vi "Parse Value.vi"(0 "JSON String":string, 5 "Index In":i32, 11 "error in (no error)":errorcluster) -> (4 "Variant out":variant, 6 "Index Out":i32, 15 "error out":errorcluster)   [LabVIEW 2017, in "Variant JSON API.lvlib"]
uses:
  Variant JSON API.lvlib
  Errors.ctl
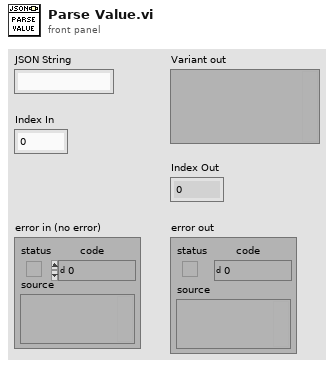
[diagram p1: front panel]
types:
  T1 = typedef "Variant JSON API.lvlib/Errors.ctl" = enum16{"No key", "Key path type", "Array OOB", "Type Mismatch", "Invalid Token", "Invalid Value"}
  T2 = typedef "Variant JSON API.lvlib/Token Type.ctl" = enum16{"NONE", "CURLY_OPEN", "CURLY_CLOSE", "SQUARED_OPEN", "SQUARED_CLOSE", "COLON", "COMMA", "STRING", "NUMBER", "TRUE", "FALSE", "NULL"}
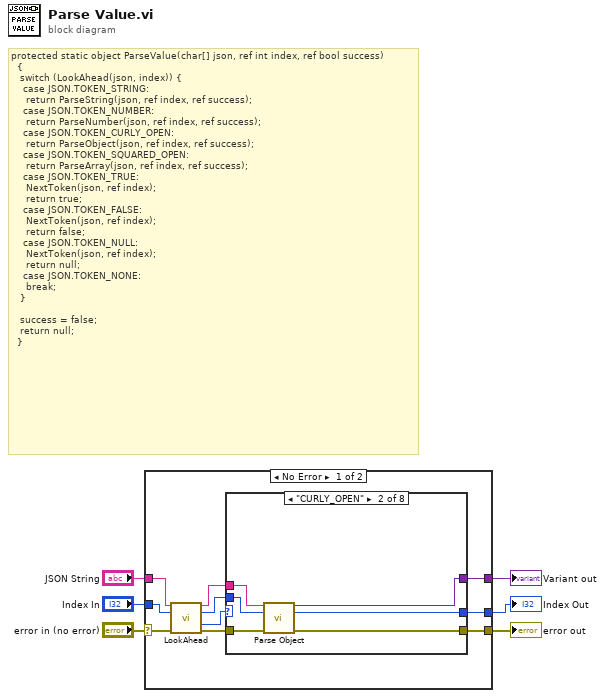
[diagram p0: block diagram]
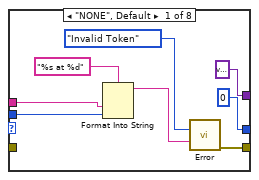
[diagram p2: hidden frame]
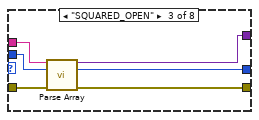
[diagram p3: hidden frame]
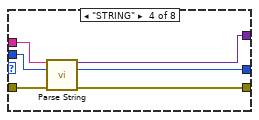
[diagram p4: hidden frame]
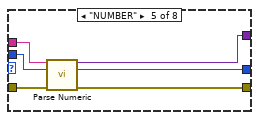
[diagram p5: hidden frame]
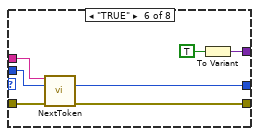
[diagram p6: hidden frame]
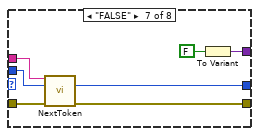
[diagram p7: hidden frame]
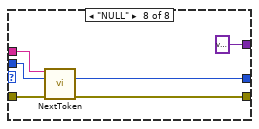
[diagram p8: hidden frame]
diagram:
  # "protected static object ParseValue(char[] json, ref int index, ref bool success)\n\t\t{\n\t\t\tswitch (LookAhead(json, index)) {\n\t\t\t\tcase JSON.TOKEN_STRING:\n\t\t\t\t\treturn ParseString(json, ref index, ref success);\n\t\t\t\tcase JSON.TOKEN_NUMBER:\n\t\t\t\t\treturn ParseNumber(json, ref index, ref success);\n\t\t\t\tcase JSON.TOKEN_CURLY_OPEN:\n\t\t\t\t\treturn ParseObject(json, ref index, ref success);\n\t\t\t\tcase JSON.TOKEN_SQUARED_OPEN:\n\t\t\t\t\treturn ParseArray(json, ref index, ref success);\n\t\t\t\tcase JSON.TOKEN_TRUE:\n\t\t\t\t\tNextToken(json, ref index);\n\t\t\t\t\treturn true;\n\t\t\t\tcase JSON.TOKEN_FALSE:\n\t\t\t\t\tNextToken(json, ref index);\n\t\t\t\t\treturn false;\n\t\t\t\tcase JSON.TOKEN_NULL:\n\t\t\t\t\tNextToken(json, ref index);\n\t\t\t\t\treturn null;\n\t\t\t\tcase JSON.TOKEN_NONE:\n\t\t\t\t\tbreak;\n\t\t\t}\n\n\t\t\tsuccess = false;\n\t\t\treturn null;\n\t\t}"
  n1 = case shown="No Error" "error in (no error)" {
    selector: "error in (no error)" -> [w16 w69]
    tunnel: [w14 w69] -> w5
    tunnel: "JSON String" -> [w10 _]
    tunnel: "Index In" -> [w9 _]
    tunnel: [w8 _] -> w1
    tunnel: [w7 _] -> w2
    frame No Error {
      n2 = call "LookAhead.vi"("JSON String"=w10, "Index"=w9, "error in (no error)"=w16) -> ("JSON String Passthrough"=w12:string, "Index Passthrough"=w11:i32, "TOKEN"=w13:T2, "error out"=w15:errorcluster)  [unwired: 9 in]
      n3 = case shown="\"CURLY_OPEN\"" w13 {
        tunnel: w15 -> [_ w28 w34 w40 w46 w52 w61 w65]
        tunnel: [w23 w27 w33 w39 w45 w51 w58 w68] -> w14
        tunnel: [variant ("Variant") w25 w31 w37 w43 w49 w56 variant ("Variant")] -> w8
        tunnel: w12 -> [w20 w29 w36 w42 w48 w55 w59 w67]
        tunnel: w11 -> [w19 w30 w35 w41 w47 w54 w60 w66]
        tunnel: [0 ("Index Out") w26 w32 w38 w44 w53 w62 w64] -> w7
        frame "NONE", Default {
          n4 = Format Into String(format string="%s at %d", w20, w19) -> (resulting string=w18:string)  [unwired: 2 in, 1 out]
          n5 = call "Error.vi"(5:Errors."Invalid Token", "Data"=w18) -> ("error out"=w23:errorcluster)  [unwired: 13 in]
        }
        frame "CURLY_OPEN" {
          n6 = call "Parse Object.vi"("JSON String"=w29, "Index In"=w30, "error in (no error)"=w28) -> ("Variant out"=w25:variant, "Index Out"=w26:i32, "error out"=w27:errorcluster)  [unwired: 10 in]
        }
        frame "SQUARED_OPEN" {
          n7 = call "Parse Array.vi"("JSON String"=w36, "Index In"=w35, "error in (no error)"=w34) -> ("Variant out"=w31:variant, "Index Out"=w32:i32, "error out"=w33:errorcluster)  [unwired: 10 in]
        }
        frame "STRING" {
          n8 = call "Parse String.vi"("JSON String"=w42, "Index In"=w41, "error in (no error)"=w40) -> ("Variant out"=w37:variant, "Index Out"=w38:i32, "error out"=w39:errorcluster)  [unwired: 9 in, 1 out]
        }
        frame "NUMBER" {
          n9 = call "Parse Numeric.vi"("JSON String"=w48, "Index In"=w47, "error in (no error)"=w46) -> ("Variant out"=w43:variant, "Index Out"=w44:i32, "error out"=w45:errorcluster)  [unwired: 10 in]
        }
        frame "TRUE" {
          n10 = call "NextToken.vi"("JSON String"=w55, "Index In"=w54, "error in (no error)"=w52) -> ("Index Out"=w53:i32, "error out"=w51:errorcluster)  [unwired: 9 in, 2 out]
          n11 = To Variant(anything=TRUE) -> (Variant=w49:variant)
        }
        frame "FALSE" {
          n12 = call "NextToken.vi"("JSON String"=w59, "Index In"=w60, "error in (no error)"=w61) -> ("Index Out"=w62:i32, "error out"=w58:errorcluster)  [unwired: 9 in, 2 out]
          n13 = To Variant(anything=FALSE) -> (Variant=w56:variant)
        }
        frame "NULL" {
          n14 = call "NextToken.vi"("JSON String"=w67, "Index In"=w66, "error in (no error)"=w65) -> ("Index Out"=w64:i32, "error out"=w68:errorcluster)  [unwired: 9 in, 2 out]
        }
      }
    }
    frame Error {
    }
  }
  "error out" <- w5
  "Index Out" <- w2
  "Variant out" <- w1
